vi "set up centrally triggered task.vi"(8 "error in":errorcluster, 9 "SampQuant.SampPerChan":dbl, 10 "source":tag, 11 "task/channels in":refnum<k21>) -> (0 "error out":errorcluster, 3 "task out":refnum<k21>)   [LabVIEW 2025]
uses:
  <resource>/objmgr/daqmx.rc
  <vilib>/DAQmx/configure/trigger.llb/DAQmx Start Trigger (Digital Edge).vi
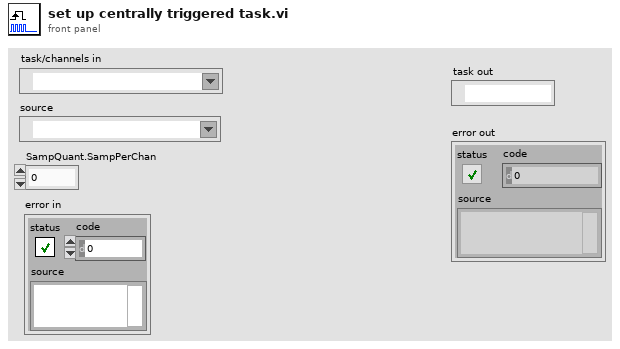
[diagram p1: front panel]
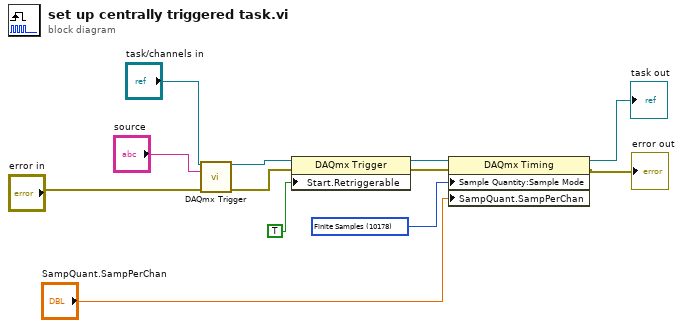
[diagram p0: block diagram]
diagram:
  w5 = 10178 items=["Finite Samples"=10178, "Continuous Samples"=10123, "Hardware Timed Single Point"=12522] ("SampQuant.SampMode")
  n1 = call-poly <vilib>:"DAQmx Trigger.vi"("task/channels in"="task/channels in", "source"="source", "error in"="error in") -> ("task out"=w12:refnum<k21>, "error out"=w10:errorcluster)  [unwired: 11 in]
  n2 = property class="DAQmx Trigger"(reference=w12, error in=w10, "Start.Retriggerable"=TRUE) -> (reference out=w11:refnum<k21>, error out=w9:errorcluster)
  n3 = property class="DAQmx Timing"(reference=w11, error in=w9, "Sample Quantity:Sample Mode"=w5, "SampQuant.SampPerChan"="SampQuant.SampPerChan") -> (reference out=→"task out":refnum<k21>, error out=→"error out":errorcluster)
